vi "Total Cycle Count.vi"(10 "Water Outlet Valve - LDO":bool, 11 "Counter of burner cycle":u16) -> (3 "Total Cycle Count":u16)   [LabVIEW 2020, in "Modbus.lvlib"]
uses:
  Modbus/Modbus.lvlib
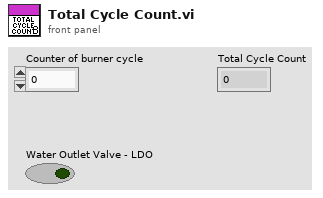
[diagram p1: front panel]
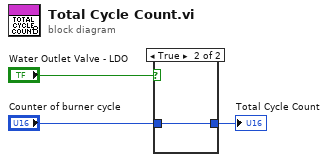
[diagram p0: block diagram]
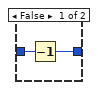
[diagram p2: hidden frame]
diagram:
  n1 = case shown="True" "Water Outlet Valve - LDO" {
    tunnel: "Counter of burner cycle" -> [w5 w6]
    tunnel: [w4 w6] -> w1
    frame False {
      n2 = Decrement(x=w5) -> (x-1=w4:u16)
    }
    frame True {
    }
  }
  "Total Cycle Count" <- w1
